vi "Get Routing and Faulting Parent Ref.vi"(8 "error in":errorcluster, 11 "routing and faulting child in":T1 format="%.0x") -> (0 "error out":errorcluster, 2 "routing and faulting":T1 format="%.0x", 3 "routing and faulting child out":T1 format="%.0x")   [LabVIEW 2020, in "Routing and Faulting Scripting.lvlib"]
uses:
  Routing and Faulting Scripting.lvlib
  <vilib>/NI VeriStand/Custom Device API/Custom Device Item Ref.ctl
  NationalInstruments.VeriStand.SystemDefinitionAPI
  NationalInstruments.VeriStand.SystemStorage
  Shared/Constants.vi
  Dependencies.llb/Routing and Faulting Shared.lvlib
  <vilib>/NI VeriStand/Custom Device API/Custom Device API.lvlib
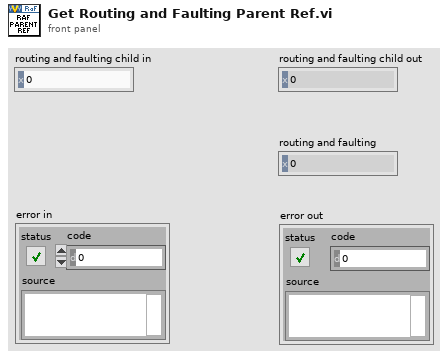
[diagram p1: front panel]
types:
  T1 = typedef "Custom Device API.lvlib/Custom Device Item Ref.ctl" = u64
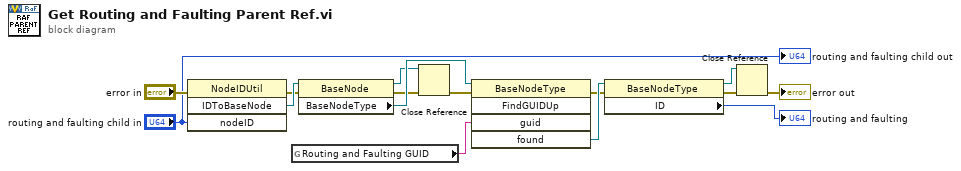
[diagram p0: block diagram]
diagram:
  n1 = invoke class="NodeIDUtil" method="IDToBaseNode"(error in="error in", "nodeID"="routing and faulting child in") -> (error out=w10:errorcluster, "IDToBaseNode"=w13:refnum<k24>)  [unwired: 2 in, 2 out]
  n2 = global read "Constants.vi" "Routing and Faulting GUID"() -> (w11:string)
  n3 = property class="BaseNode"(reference=w13, error in=w10) -> (reference out=w6:refnum<k24>, error out=w7:errorcluster, "BaseNodeType"=w12:refnum<k24>)
  n4 = Close Reference(reference=w6, error in (no error)=w7) -> (error out=w5:errorcluster)
  n5 = invoke class="BaseNodeType" method="FindGUIDUp"(reference=w12, error in=w5, "guid"=w11) -> (error out=w8:errorcluster, "found"=w9:refnum<k24>)  [unwired: 2 in, 3 out]
  n6 = property class="BaseNodeType"(reference=w9, error in=w8) -> (reference out=w2:refnum<k24>, error out=w4:errorcluster, "ID"=→"routing and faulting":u64)
  n7 = Close Reference(reference=w2, error in (no error)=w4) -> (error out=→"error out":errorcluster)
  "routing and faulting child out" <- "routing and faulting child in"
